vi "FRCts20_EspEngine_RequestsPerHour_Line.vi"(8 "error in (no error)":errorcluster, 10 "RequestsPerHour":T1, 11 "httpRequestID":u32) -> (0 "error out":errorcluster, 3 "httpRequestID out":u32)   [LabVIEW 2013, in "FRCts20_EspEngine.lvlib"]
uses:
  FRCts20_EspEngine.lvlib
  TypeDefs/FRCts20_EspEngine_RequestPerHour_Line.ctl
  <vilib>/wsapi/subVIs/Set Integer ESP Variable.vi
  FRCts20_EspEngine_FormatArrayOfKeysStrings.vi
  <vilib>/wsapi/NI_WebServices.lvlib
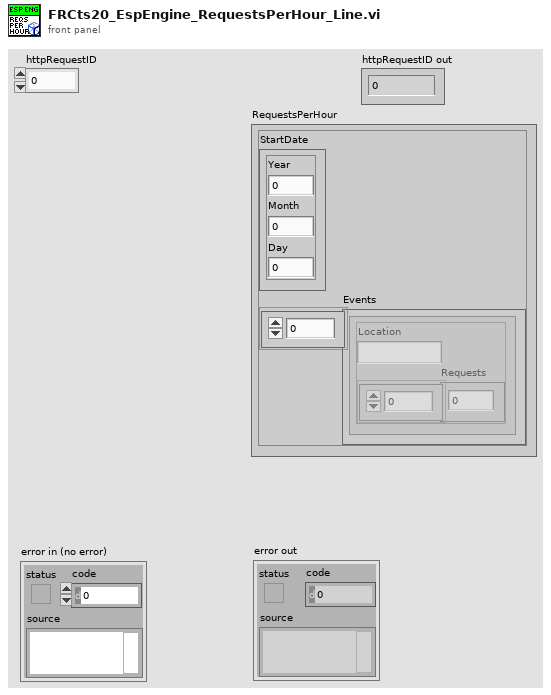
[diagram p1: front panel]
types:
  T1 = typedef "FRCts20_EspEngine.lvlib/FRCts20_EspEngine_RequestPerHour_Line.ctl" = cluster{"StartDate":cluster{"Year":i32, "Month":i32, "Day":i32}, "Events":cluster{"Location":string, "Requests":i32[]}[]}
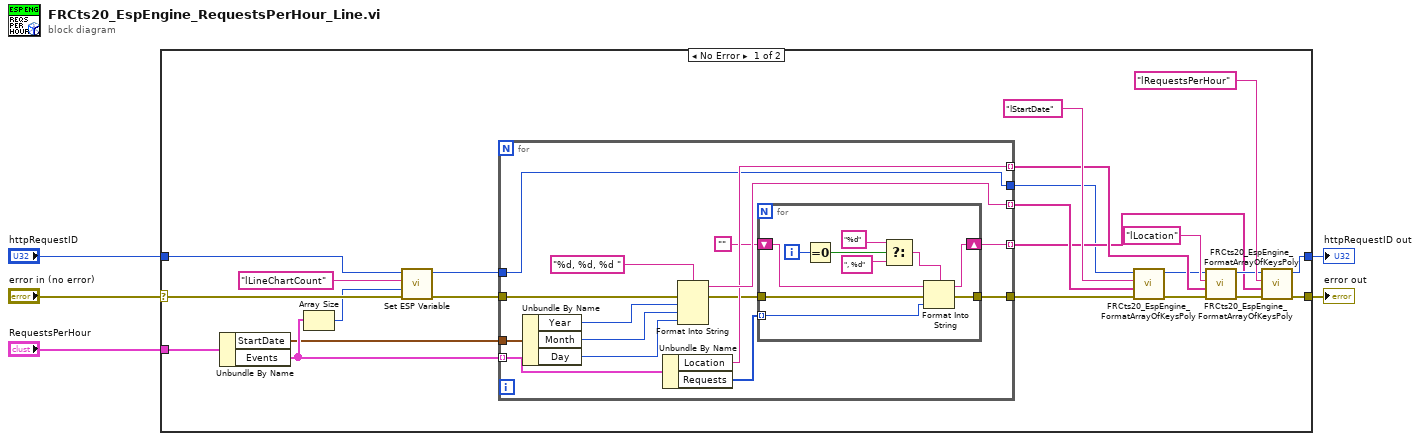
[diagram p0: block diagram]
diagram:
  n1 = case shown="No Error" "error in (no error)" {
    selector: "error in (no error)" -> [w26 w55]
    tunnel: [w10 w55] -> w5
    tunnel: "httpRequestID" -> [w27 w54]
    tunnel: "RequestsPerHour" -> [w24 _]
    tunnel: [w9 w54] -> w1
    frame No Error {
      n2 = Unbundle By Name(w24) -> ("StartDate"=w22:cluster{"Year":i32, "Month":i32, "Day":i32}, "Events"=w23:cluster{"Location":string, "Requests":i32[]}[])
      n3 = Array Size(array=w23) -> (size(s)=w25:i32)
      n4 = call-poly <vilib>:"Set ESP Variable.vi"("error in (no error)"=w26, "value"=w25, "key"="lLineChartCount", "httpRequestID"=w27) -> ("error out"=w19:errorcluster, "httpRequestID out"=w13:u32)  [unwired: 6 in]
      n5 = for {
        tunnel: w23 -> [w43] mode=indexing
        tunnel: w22 -> [w42]
        tunnel: [w37] -> w21 mode=indexing
        tunnel: w19 -> [w36]
        tunnel: [w35] -> w18 mode=indexing
        tunnel: w13 -> [w30]
        tunnel: [w32] -> w8 mode=indexing
        tunnel: [w31] -> w7
        tunnel: [w30] -> w6
        n6 = Unbundle By Name(w42) -> ("Year"=w40:i32, "Month"=w39:i32, "Day"=w38:i32)
        n7 = Unbundle By Name(w43) -> ("Location"=w35:string, "Requests"=w34:i32[])
        n8 = Format Into String(format string="%d, %d, %d ", error in=w36, w40, w39, w38) -> (resulting string=w37:string, error out=w33:errorcluster)  [unwired: 1 in]
        n9 = for {
          tunnel: w34 -> [w52] mode=indexing
          tunnel: w33 -> [w53]
          shift-right: [w51] -> w32
          shift-left: "" -> [w50]
          tunnel: [w44] -> w31
          i -> [w49]
          n10 = Equal To 0?(x=w49) -> (x = 0?=w48:bool)
          n11 = Select(t="%d", s=w48, f=", %d" ("format string")) -> (s? t:f=w45:string)
          n12 = Format Into String(format string=w45, initial string=w50, error in=w53, w52) -> (resulting string=w51:string, error out=w44:errorcluster)
        }
      }
      n13 = call-poly "FRCts20_EspEngine_FormatArrayOfKeysPoly.vi"("error IO"=w7, "Values"=w21, "KeyBaseName"="lStartDate", "httpRequestID"=w6) -> ("error IO"=w16:errorcluster, "httpRequestID out"=w12:u32)  [unwired: 6 in]
      n14 = call-poly "FRCts20_EspEngine_FormatArrayOfKeysPoly.vi"("error IO"=w16, "Values"=w18, "KeyBaseName"="lLocation", "httpRequestID"=w12) -> ("error IO"=w14:errorcluster, "httpRequestID out"=w11:u32)  [unwired: 6 in]
      n15 = call-poly "FRCts20_EspEngine_FormatArrayOfKeysPoly.vi"("error IO"=w14, "Values"=w8, "KeyBaseName"="lRequestsPerHour", "httpRequestID"=w11) -> ("error IO"=w10:errorcluster, "httpRequestID out"=w9:u32)  [unwired: 6 in]
    }
    frame Error {
    }
  }
  "error out" <- w5
  "httpRequestID out" <- w1
